vi "Virtual shutter enable disable.vi"(8 "error in (no error)":errorcluster, 9 "Cancelled":bool, 11 "Virtual Shutter":T1) -> (0 "error out":errorcluster)   [LabVIEW 2013]
uses:
  Typedefs/Shutter state.ctl
  Global Variables/gl_UI Ctrl Refs.vi
  Global Variables/General Globals.vi
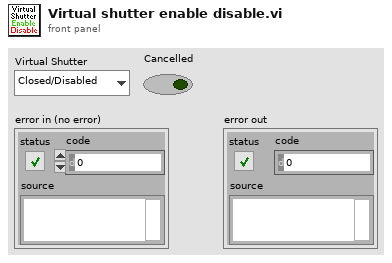
[diagram p1: front panel]
types:
  T1 = typedef "Shutter state.ctl" = enum16{"Closed/Disabled", "Open/Enabled"}
  T2 = typedef "UI ctrl refs cluster.ctl" = cluster{"Top level VI path":path, "Top level VI ref":refnum<vi>, "User menu ref":refnum<k9>, "Sub Panel control":refnum<vi>, "Imaging Param Tab":refnum<vi>, "Occurrence-Start drivers":refnum<k4>, "Occurrence-Speed logging initialised":refnum<k4>, "Occurrence-XYZ stage initialised":refnum<k4>, "Exit button":refnum<vi>, "Status ind":refnum<vi>, "Return to Origin":refnum<vi>, "Speed Logging":refnum<vi>, "Time Lapse":refnum<vi>, "Live Imaging":refnum<vi>, "AOL Z Stack":refnum<vi>, "Motor Z Stack":refnum<vi>, "Funct Acq button":refnum<vi>, "Hard Shutter":refnum<vi>, "Virtual Shutter":refnum<vi>, "Laser Power":refnum<vi>, "AOL Mode":refnum<vi>, "Frame Size":refnum<vi>, "Field of View":refnum<vi>, "Dwell Time":refnum<vi>, "Zoom":refnum<vi>, "AOL Z":refnum<vi>, "Objective":refnum<vi>, "Axis":refnum<vi>, "Paths & Names":refnum<vi>, "Experiment folder path (ind.)":refnum<vi>, "Last State (Ind.)":refnum<vi>, "Laser wavelength ind (nm)":refnum<vi>, "Averages":refnum<vi>, "Angle (degrees)":refnum<vi>, "X centre":refnum<vi>, "Y centre":refnum<vi>, "Plane Mode":refnum<vi>, "# Planes":refnum<vi>, "Z Start":refnum<vi>, "Z Stop":refnum<vi>, "Z Step":refnum<vi>, "PMT 1":refnum<vi>, "PMT 2":refnum<vi>, "Stage XYZ Position":refnum<vi>, "Pockels@Z Start":refnum<vi>, "Pockels@Z Stop":refnum<vi>, "Obtain Z Start":refnum<vi>, "Obtain Z Stop":refnum<vi>, "Live stim.trig.period":refnum<vi>, "Live stim.trig.enable":refnum<vi>, "Funct. Acq. Pockels Modulation":refnum<vi>, "Enable Video Recording":refnum<vi>, "Video Record-Live Imaging":refnum<vi>, "Video Record-Funct acq":refnum<vi>, "AOL Z-stack Chirps Ready (ind)":refnum<vi>, "Center freq ind (nm)":refnum<vi>, "Logging queue (ind)":refnum<vi>, "Back aperture power (ind.)":refnum<vi>, "Power after objective (ind.)":refnum<vi>, "Switch user":refnum<vi>}
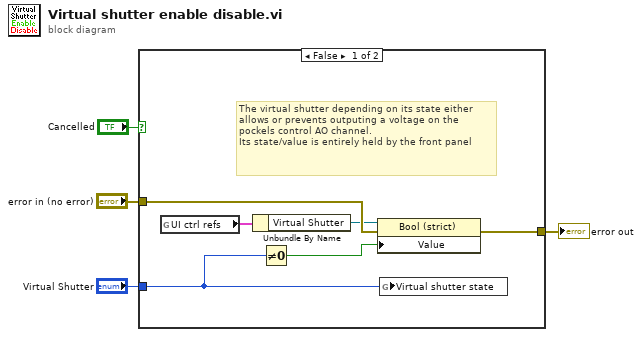
[diagram p0: block diagram]
diagram:
  n1 = case shown="False" "Cancelled" {
    tunnel: "error in (no error)" -> [w10 w11]
    tunnel: [w9 w11] -> w1
    tunnel: "Virtual Shutter" -> [w6 _]
    frame False {
      # "The virtual shutter depending on its state either allows or prevents outputing a voltage on the pockels control AO channel.\nIts state/value is entirely held by the front panel"
      n2 = global read "gl_UI Ctrl Refs.vi" "UI ctrl refs"() -> (w5:T2)
      n3 = Unbundle By Name(w5) -> ("Virtual Shutter"=w8:refnum<vi>)
      n4 = Not Equal To 0?(x=w6) -> (x != 0?=w7:bool)
      n5 = property on="Property Node" class="Bool (strict)"(reference=w8, error in=w10, "Value"=w7) -> (error out=w9:errorcluster)  [unwired: 1 out]
      n6 = global write "General Globals.vi" "Virtual shutter state"(w6) -> ()
    }
    frame True {
      # "Cancelled"
    }
  }
  "error out" <- w1
